vi "SetTrigger.vi"(8 "error in":errorcluster, 9 "ParameterLabel":string, 10 "Arg":string, 11 "Highland T564 DDG in":refnum<class "Highland T564 DDG.lvclass">) -> (0 "error out":errorcluster, 3 "Highland T564 DDG out":refnum<class "Highland T564 DDG.lvclass">)   [LabVIEW 2013, in "Highland T564 DDG.lvclass"]
uses:
  Highland T564 DDG.lvclass
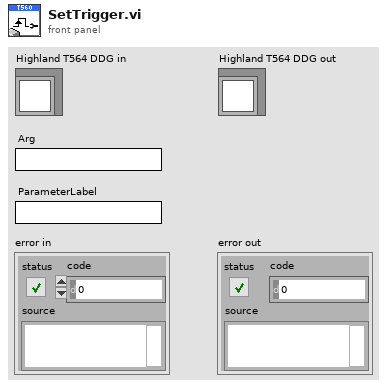
[diagram p1: front panel]
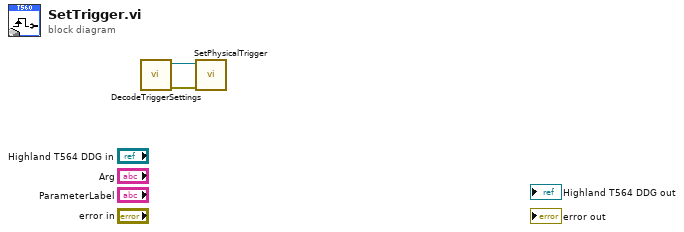
[diagram p0: block diagram]
diagram:
  n1 = call-dynamic "DecodeTriggerSettings.vi"() -> ("error out"=w2:errorcluster, "Highland T564 DDG out"=w1:refnum<class "Highland T564 DDG.lvclass">)  [unwired: 10 in]
  n2 = call-dynamic "SetPhysicalTrigger.vi"("error in (no error)"=w2, "Highland T564 DDG in"=w1) -> ()  [unwired: 8 in, 2 out]
